vi "MPExxx Query Register.vi"(3 "error in (no error)":errorcluster {"code" format="%.0x"}, 4 "Register Query":u8(ring) items=["Event Status Enable", "Event Staus", "Service Request Enable", "Status Byte"], 5 "VISA session":refnum<visa-resource-name>) -> (0 "error out":errorcluster {"code" format="%.0x"}, 1 "Value":string, 2 "dup VISA session":refnum<visa-resource-name>)   [LabVIEW 2012]
doc: "Queries the power supply's register values."
panel:
  # "MAGNA-POWER"
  # "Electronics"
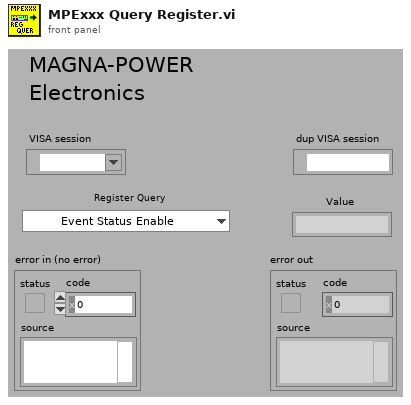
[diagram p1: front panel]
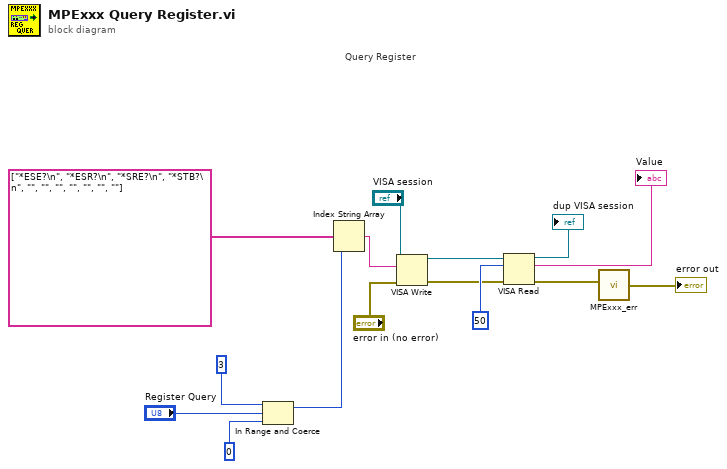
[diagram p0: block diagram]
diagram:
  # "Query Register"
  n1 = In Range and Coerce(upper limit=3, x="Register Query", lower limit=0) -> (coerced(x)=w1:i32)  [unwired: 1 out]
  n2 = Index String Array(1:w1, 2:string[] ["*ESE?\n", "*ESR?\n", "*SRE?\n", "*STB?\n", "", "", "", "", "", "", ""] ("Array Constant")) -> (0:w12:string)  [unwired: 1 in]
  n3 = VISA Write(VISA resource name="VISA session", write buffer=w12, error in (no error)="error in (no error)") -> (VISA resource name out=w10:refnum<visa-resource-name>, error out=w9:errorcluster)  [unwired: 1 out]
  n4 = VISA Read(VISA resource name=w10, byte count=u32 50 ("byte count (0)"), error in (no error)=w9) -> (VISA resource name out=→"dup VISA session":refnum<visa-resource-name>, read buffer=→"Value":string, error out=w7:errorcluster)  [unwired: 1 out]
  n5 = call "MPExxx_err.vi"("error in (no error)"=w7) -> ("error out"=→"error out":errorcluster)
